vi "SetParam.vi"(8 "error in (no error)":errorcluster caption="entrée d'erreur (pas d'erreur)", 10 "HashingVectorizer":T1={"encoding"="utf-8", "decode_error"="strict", "strip_accents"="None", "lowercase"=TRUE, "preprocessor"="None", "tokenizer"="None", "stop_words"={"Type"="None", "list"=[]}, "token_pattern"="(?u)\\b\\w\\w+\\b", "ngram_range"={"min_n"=1, "max_n"=1}, "analyzer"="word", "n_features"=1048576, "binary"=FALSE, "norm"="l2", "alternate_sign"=TRUE, "dtype"="float"}, 11 "HashingVectorizer.lvclass":refnum<class "HashingVectorizer.lvclass">) -> (0 "error out":errorcluster caption="sortie d'erreur", 3 "HashingVectorizer.lvclass":refnum<class "HashingVectorizer.lvclass">)   [LabVIEW 2020, in "HashingVectorizer.lvclass"]
doc: "Set Parameters"
uses:
  HashingVectorizer.lvclass
  HashingVectorizer.lvclass/HashingVectorizer.ctl
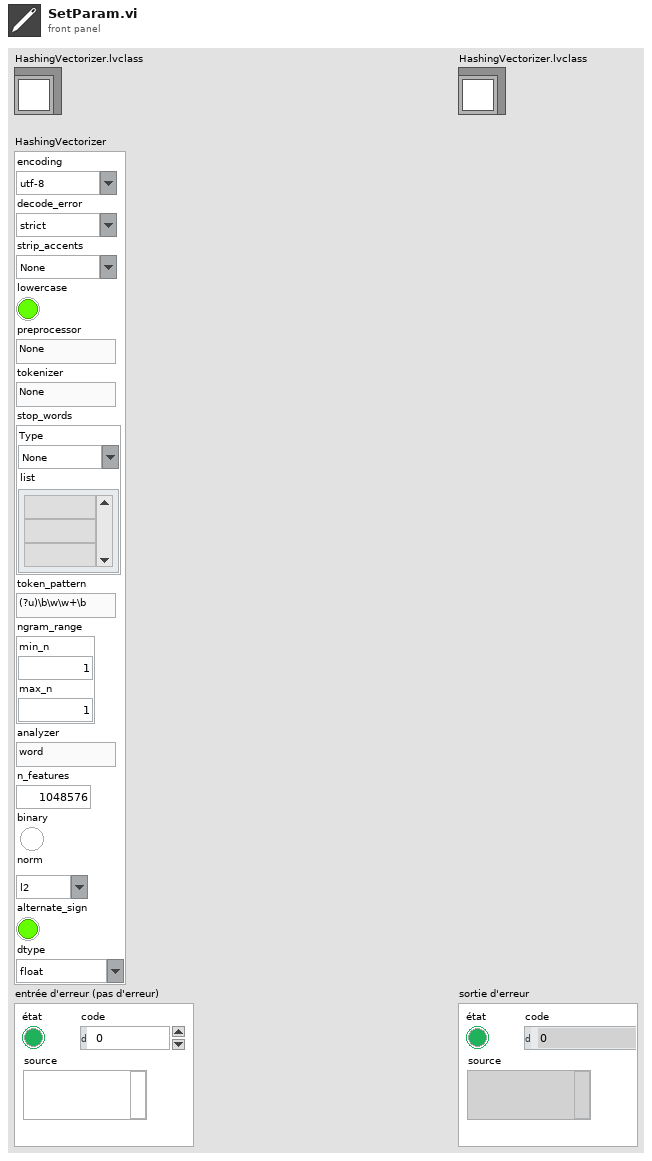
[diagram p1: front panel]
types:
  T1 = cluster{"encoding":string, "decode_error":string, "strip_accents":string, "lowercase":bool, "preprocessor":string, "tokenizer":string, "stop_words":cluster{"Type":string, "list":string[]}, "token_pattern":string, "ngram_range":cluster{"min_n":i32, "max_n":i32}, "analyzer":string, "n_features":i32, "binary":bool, "norm":string, "alternate_sign":bool, "dtype":string}
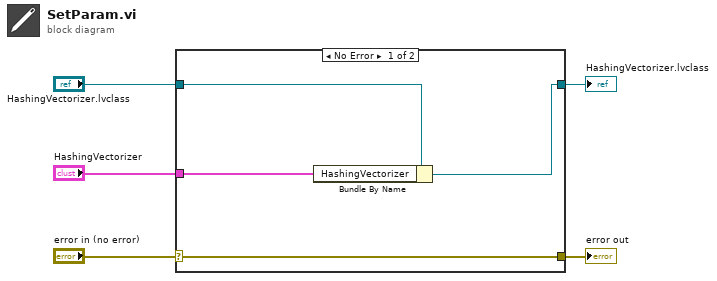
[diagram p0: block diagram]
diagram:
  n1 = case shown="No Error" "error in (no error)" {
    selector: "error in (no error)" -> [w9 w10]
    tunnel: [w9 w10] -> w4
    tunnel: [w7 w11] -> w2
    tunnel: "HashingVectorizer.lvclass" -> [w8 w11]
    tunnel: "HashingVectorizer" -> [w6 _]
    frame No Error {
      n2 = Bundle By Name(cluster=w8, "HashingVectorizer"=w6) -> (w7:refnum<class "HashingVectorizer.lvclass">)
    }
    frame Error {
    }
  }
  "error out" <- w4
  "HashingVectorizer.lvclass" <- w2
